vi "Configure Resistivity.vi"(5 "User Resistivity Type (0: Surface)":i32(ring) items=["Surface", "Volume"], 6 "User Kv Volume Resistivity (2.290000E+1)":dbl=22.9 format="%.6e", 7 "User Ks Surface Resistivity (5.340000E+1)":dbl=53.4 format="%.6e", 8 "error in (no error)":errorcluster, 9 "Volume Resistivity Sample Thickness (1.000000E+0)":dbl=1.0 format="%.6e", 10 "Test Fixture (1: USER)":i32(ring)=1 items=["M8009", "USER"], 11 "VISA resource name":refnum<visa-resource-name>) -> (0 "error out":errorcluster, 3 "VISA resource name out":refnum<visa-resource-name>)   [LabVIEW 2020, in "Keithley 6517.lvlib"]
doc: "Configures resistivity measurements, including test fixture type, sample thickness for volume resistivity, measurement type for the user test fixture, Ks parameter for surface resistivity and Kv parameter for volume resistivity.\n\nNote:\nResistance measurement should be enabled from <b>Configure Measurement Function.vi</b>.\n\nThis VI is <B>NOT</B> compatible with model <B>6514</B>."
uses:
  <instrlib>/Keithley 6517/Keithley 6517.lvlib
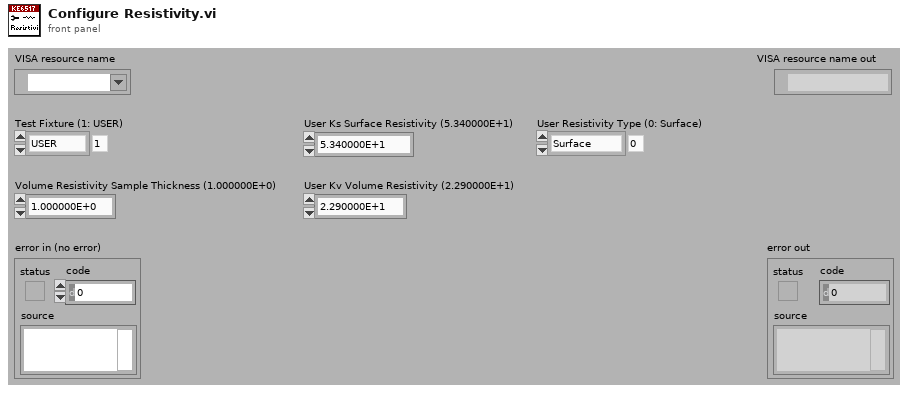
[diagram p1: front panel]
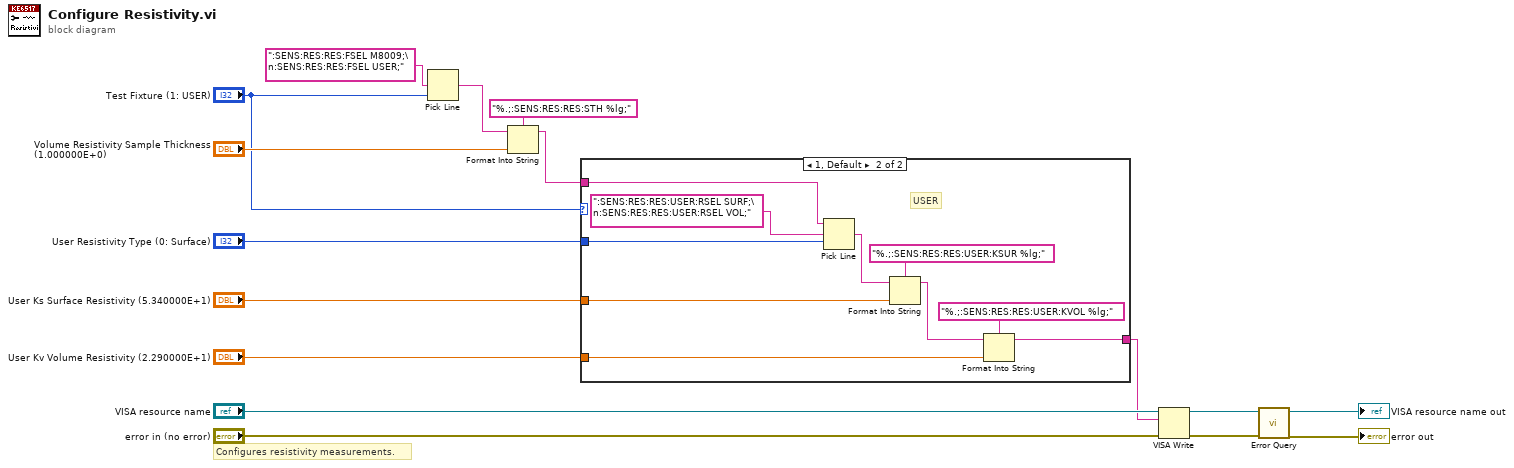
[diagram p0: block diagram]
diagram:
  # "Configures resistivity measurements."
  n1 = Pick Line(multi-line string=":SENS:RES:RES:FSEL M8009;\n:SENS:RES:RES:FSEL USER;", line index="Test Fixture (1: USER)") -> (output string=w7:string)  [unwired: 1 in]
  n2 = Format Into String(format string="%.;:SENS:RES:RES:STH %lg;", initial string=w7, "Volume Resistivity Sample Thickness (1.000000E+0)") -> (resulting string=w1:string)  [unwired: 1 in, 1 out]
  n3 = case shown="1, Default" "Test Fixture (1: USER)" {
    tunnel: "User Resistivity Type (0: Surface)" -> [_ w22]
    tunnel: "User Ks Surface Resistivity (5.340000E+1)" -> [_ w21]
    tunnel: "User Kv Volume Resistivity (2.290000E+1)" -> [_ w20]
    tunnel: [w17 w19] -> w2
    tunnel: w1 -> [w17 w18]
    frame 0 {
      # "M8009, nothing to do here."
    }
    frame 1, Default {
      # "USER"
      n4 = Pick Line(string ("")=w18, multi-line string=":SENS:RES:RES:USER:RSEL SURF;\n:SENS:RES:RES:USER:RSEL VOL;", line index=w22) -> (output string=w27:string)
      n5 = Format Into String(format string="%.;:SENS:RES:RES:USER:KSUR %lg;", initial string=w27, w21) -> (resulting string=w24:string)  [unwired: 1 in, 1 out]
      n6 = Format Into String(format string="%.;:SENS:RES:RES:USER:KVOL %lg;", initial string=w24, w20) -> (resulting string=w19:string)  [unwired: 1 in, 1 out]
    }
  }
  n7 = VISA Write(VISA resource name="VISA resource name", write buffer=w2, error in (no error)="error in (no error)") -> (VISA resource name out=w12:refnum<visa-resource-name>, error out=w11:errorcluster)  [unwired: 1 out]
  n8 = call <instrlib>:"Error Query.vi"("error in (no error)"=w11, "VISA resource name"=w12) -> ("error out"=→"error out":errorcluster, "VISA resource name out"=→"VISA resource name out":refnum<visa-resource-name>)  [unwired: 6 in, 2 out]
